vi "Overflow.vi"(10 "Limit":dbl=1.0 format="%#_13g", 11 "Value":dbl format="%#_13g") -> (3 "Overflow":dbl)   [LabVIEW 2019]
doc: "This VI calculates the overflow of an input."
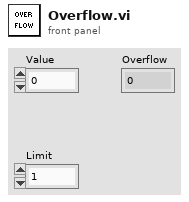
[diagram p1: front panel]
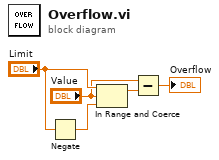
[diagram p0: block diagram]
diagram:
  n1 = Negate(x="Limit") -> (-x=w5:dbl)
  n2 = In Range and Coerce(upper limit="Limit", x="Value", lower limit=w5) -> (coerced(x)=w3:dbl)  [unwired: 1 out]
  n3 = Subtract(x="Value", y=w3) -> (x-y=→"Overflow":dbl)
